vi "play_Test_observer.vi"() -> ()   [LabVIEW 2017]
uses:
  <vilib>/FPGAPlugInAG/cRIO-9082/niLvFpga_Open_cRIO-9082.vi
  <vilib>/rvi/interface/common/dynamic/niFpgaDynamicAddResources.vi
  <vilib>/FPGAPlugInAG/Dynamic/niLvFpga_Reset_Dynamic.vi
  <vilib>/rvi/interface/common/niFpgaWaitOnOcc.vi
  <vilib>/Utility/error.llb/Error Cluster From Error Code.vi
  <vilib>/rvi/errors/niLvFpgaAdjustHostInterfaceError.vi
  <vilib>/FPGAPlugInAG/Dynamic/niLvFpga_Run_Dynamic.vi
  <vilib>/FPGAPlugInAG/Dynamic/niLvFpga_Close_Dynamic.vi
  <vilib>/rvi/interface/nirviOpenFPGA/nirviOpenFPGA.xnode
  FPGA Bitfiles/XYpeizocontrol_FPGATargetSPARTA_Testobserver_hvOqpVtTGOI.lvbitx
  <vilib>/rvi/interface/nirviMethod/nirviMethod.xnode
  <vilib>/rvi/interface/nirviReadWriteControl/nirviReadWriteControl.xnode
  <vilib>/rvi/interface/nirviCloseFPGA/nirviCloseFPGA.xnode
  <vilib>/rvi/errors/niLvFpgaMergeErrorWithErrorCode.vi
  <vilib>/rvi/interface/Simulation/niFpgaSimulationCallBeginRW.vi
  <vilib>/FPGAPlugInAG/Dynamic/niLvFpga_ConfigureFifo_Dynamic.vi
  <vilib>/FPGAPlugInAG/Dynamic/niLvFpga_WriteFifo_Dynamic.vi
  NiFpgaLv.dll
panel:
  in  "N_iters":i32
  in  "u(k)":sgl
  in  "y(k)":sgl
  in  "x^(k)":sgl[](array[numeric])=[0.0, 0.0, 0.0, 0.0, 0.0, 0.0, 0.0, 0.0, 0.0, 0.0, 0.0, 0.0, 0.0, 0.0, 0.0, 0.0, 0.0, 0.0, 0.0, 0.0, 0.0, 0.0, 0.0, 0.0, 0.0]
  out "x^(k+1) = Ax + Bu + Lye":sgl[](array[numeric])
  in  "Control Parameters path":path=path "C:/Users/arnold/Documents/MATLAB/AFM_SS/data/exp01Controls.csv"
  in  "Boolean":bool=TRUE
  out "Iter":i32
  out "error constant":errorcluster
  out "Depth":i32
  out "Elements Remaing":i32
  out "NS":i32
  out "output array":dbl[](array[numeric])
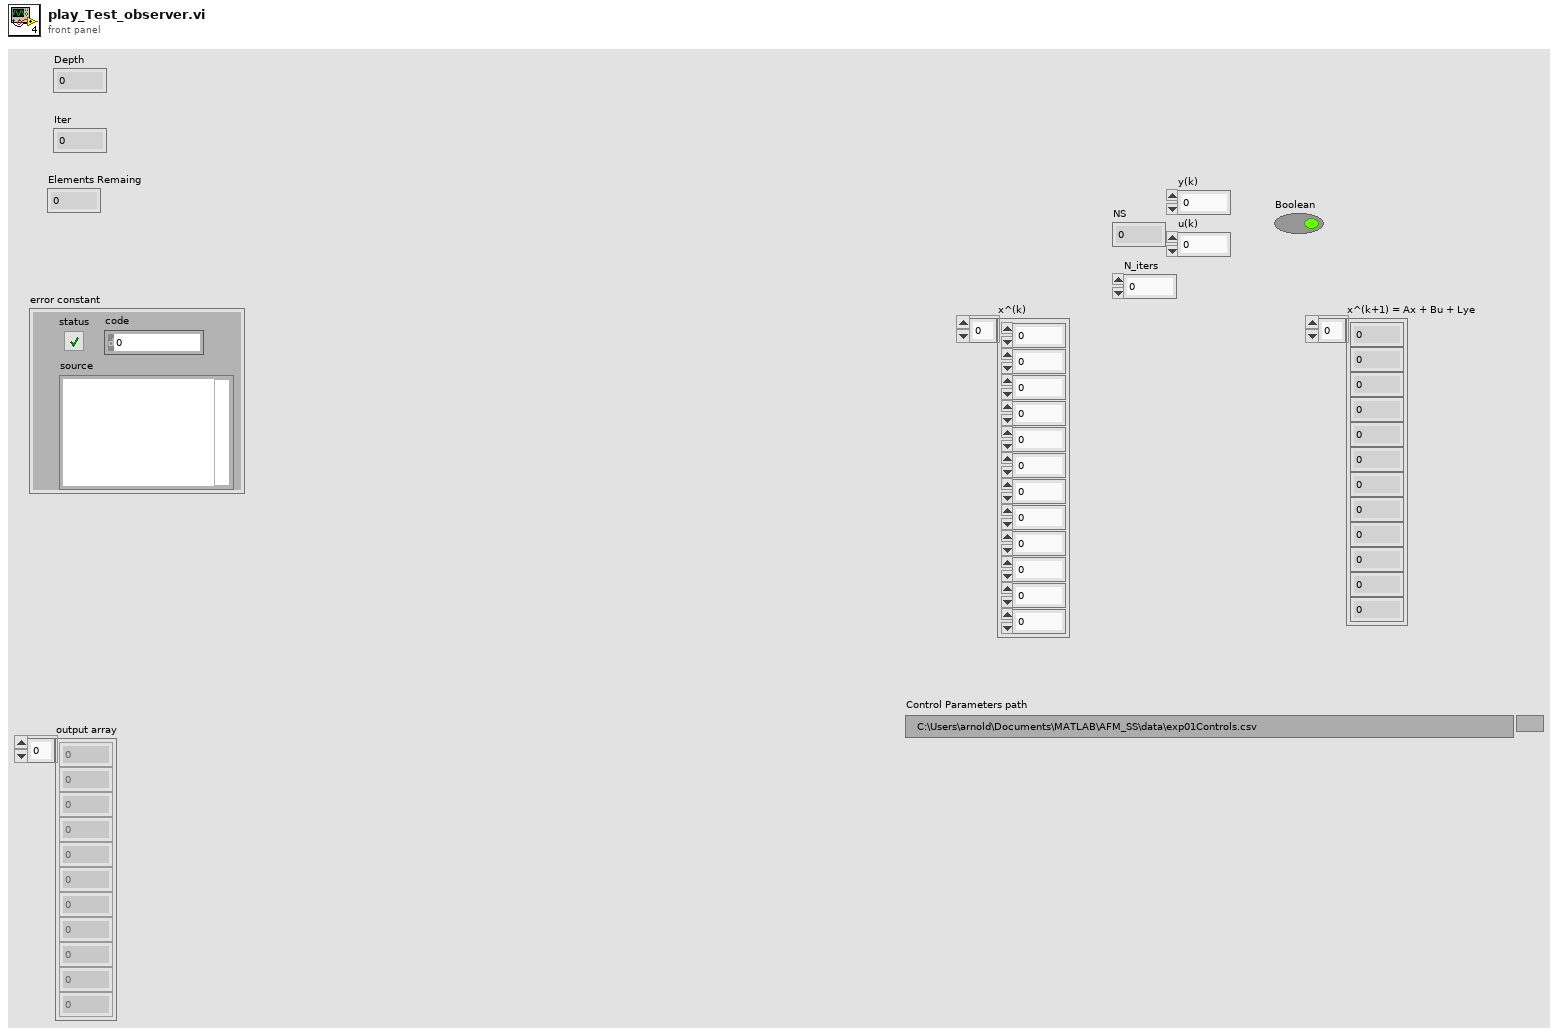
[diagram p1: front panel]
types:
  T1 = typedef "ControlParams.ctl" = cluster{"NS":i32, "ND":i32, "Nbar":dbl, "Ki":dbl, "ref":dbl}
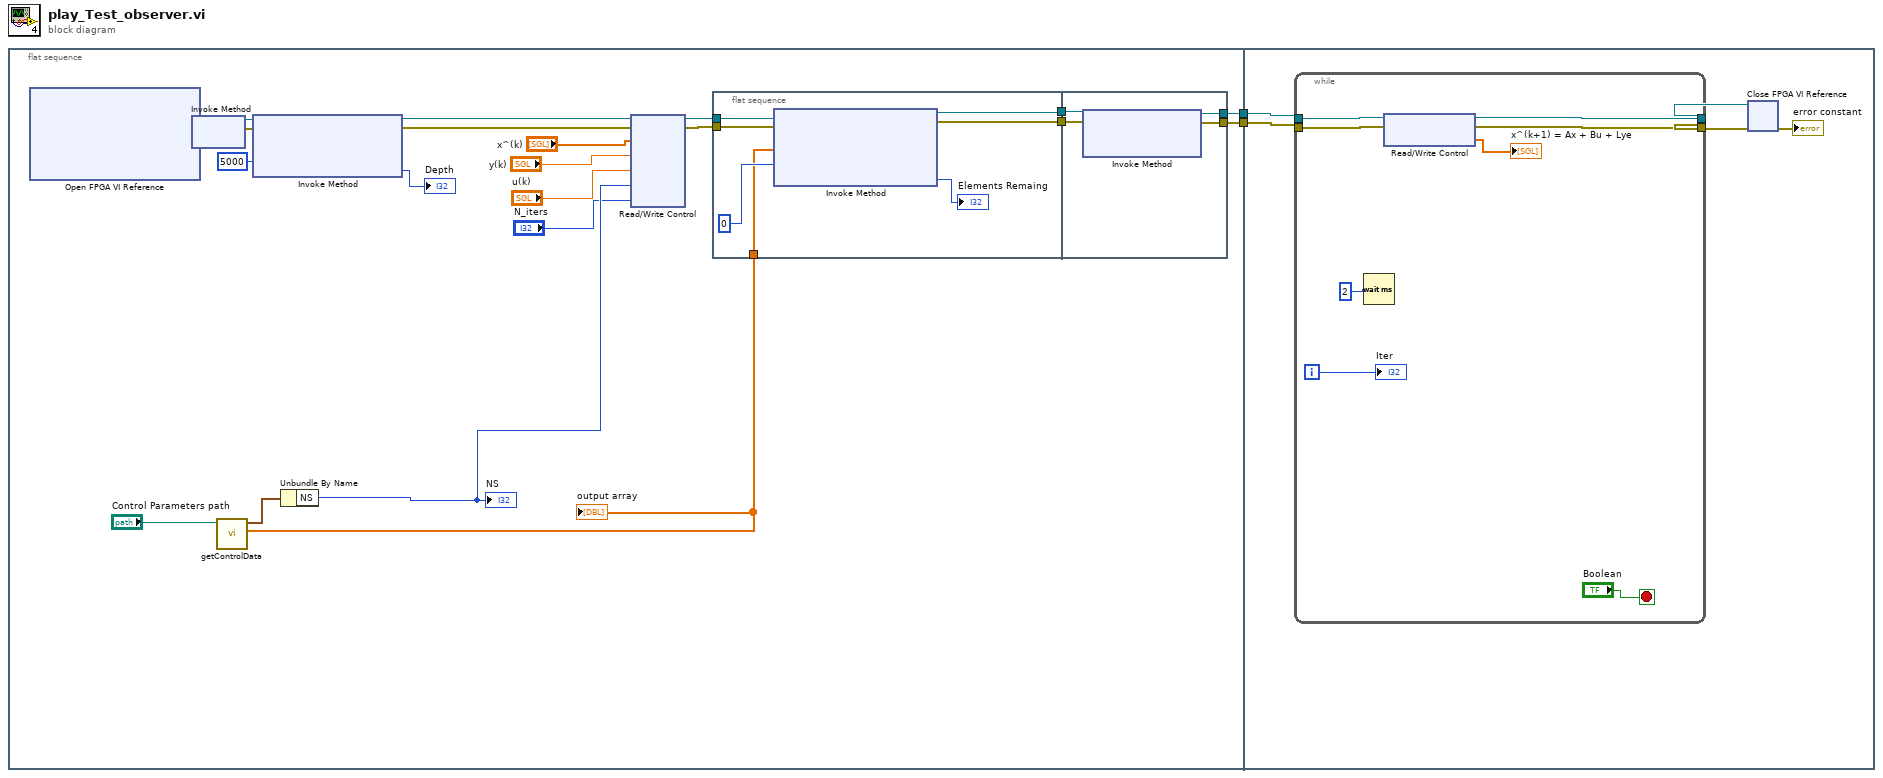
[diagram p0: block diagram]
diagram:
  n1 = flat-sequence {
    tunnel: [w16] -> w2
    tunnel: [w15] -> w1
    tunnel: w2 -> [w39]
    tunnel: w1 -> [w38]
    frame #0 {
      n2 = xnode "Open FPGA VI Reference"() -> ("FPGA VI Reference Out"=w20:refnum<k20>, "error out"=w21:errorcluster)  [unwired: 2 in]
      n3 = xnode "Invoke Method"("FPGA VI Reference In"=w20, "error in"=w21) -> ("FPGA VI Reference Out"=w23:refnum<k20>, "error out"=w24:errorcluster)
      n4 = call "getControlData.vi"("system matricec path"="Control Parameters path") -> ("AllMatrix"=w8:dbl[], "controlParams"=w9:T1)  [unwired: 9 in]
      "output array" <- w8
      n5 = xnode "Invoke Method"("FPGA VI Reference In"=w23, "error in"=w24, "Requested Depth"=5000) -> ("FPGA VI Reference Out"=w14:refnum<k20>, "error out"=w13:errorcluster, "Actual Depth"=→"Depth":u32)
      n6 = Unbundle By Name(w9) -> ("NS"=w6:i32)
      "NS" <- w6
      n7 = xnode "Read/Write Control"("FPGA VI Reference In"=w14, "error in"=w13, "X"="x^(k)", "y(k)"="y(k)", "u(k)"="u(k)", "NS"=w6, "N_iters"="N_iters") -> ("FPGA VI Reference Out"=w18:refnum<k20>, "error out"=w17:errorcluster)
      n8 = flat-sequence {
        tunnel: w8 -> [w30]
        tunnel: w18 -> [w29]
        tunnel: w17 -> [w28]
        tunnel: [w27] -> w12
        tunnel: [w26] -> w11
        tunnel: w12 -> [w35]
        tunnel: w11 -> [w34]
        tunnel: [w33] -> w16
        tunnel: [w32] -> w15
        frame #0 {
          n9 = xnode "Invoke Method"("FPGA VI Reference In"=w29, "error in"=w28, "Data"=w30, "Timeout (ms)"=0) -> ("FPGA VI Reference Out"=w27:refnum<k20>, "error out"=w26:errorcluster, "Empty Elements Remaining"=→"Elements Remaing":u32)
        }
        frame #1 {
          n10 = xnode "Invoke Method"("FPGA VI Reference In"=w35, "error in"=w34) -> ("FPGA VI Reference Out"=w33:refnum<k20>, "error out"=w32:errorcluster)  [unwired: 1 in]
        }
      }
    }
    frame #1 {
      n11 = while {
        tunnel: [w43] -> w36
        tunnel: [w42] -> w37
        tunnel: w39 -> [w45]
        tunnel: w38 -> [w44]
        i -> [w48]
        stop <- "Boolean" stop-if-true
        n12 = Wait (ms)(milliseconds to wait=2) -> ()  [unwired: 1 out]
        n13 = xnode "Read/Write Control"("FPGA VI Reference In"=w45, "error in"=w44) -> ("FPGA VI Reference Out"=w43:refnum<k20>, "error out"=w42:errorcluster, "Ax + Bu + Lye"=→"x^(k+1) = Ax + Bu + Lye":sgl[])
        "Iter" <- w48
      }
      n14 = xnode "Close FPGA VI Reference"("FPGA VI Reference In"=w36, "error in"=w37) -> ("error out"=→"error constant":errorcluster)
    }
  }
